vi "MATLAB storage.vi"   [LabVIEW 2022 SP3]
uses:
  <vilib>/Platform/storage/lvStorage.llb/xStorage/Open Data Storage/Open Data Storage.xnode
  <vilib>/Platform/storage/lvStorage.llb/_openStorageWithRootAutoDetect.vi
  <vilib>/Platform/storage/lvStorage.llb/_openFunction.ctl
  <vilib>/Platform/storage/lvStorage.llb/_defaultFilePath.vi
  <vilib>/Platform/storage/lvStorage.llb/xStorage/xStorageSupp/ErrorOut.vi
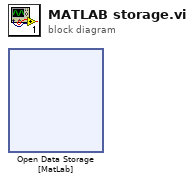
[diagram p0: block diagram]
diagram:
  n1 = xnode "Open Data Storage\n[MatLab]"() -> ()  [unwired: 5 in, 3 out]
